vi "Get Component by Unique Name.vi"(0 "Build Analyzer in":refnum<class "Build Analyzer.lvclass">, 5 "Component's Unique Name":string, 11 "error in (no error)":errorcluster) -> (4 "Build Analyzer out":refnum<class "Build Analyzer.lvclass">, 6 "Component":refnum<class "Component.lvclass">, 8 "Found":bool, 15 "error out":errorcluster)   [LabVIEW 2017, in "CL_G3_VIComponentBuilder.lvlib" / "Build Analyzer.lvclass"]
doc: "Returns a component by its unique name."
uses:
  Build Analyzer.lvclass
  Components/Component.lvclass
  Build Analyzer.lvclass/Build Analyzer.ctl
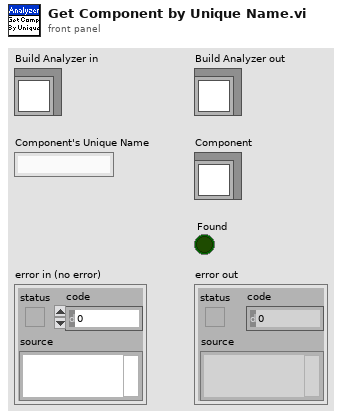
[diagram p1: front panel]
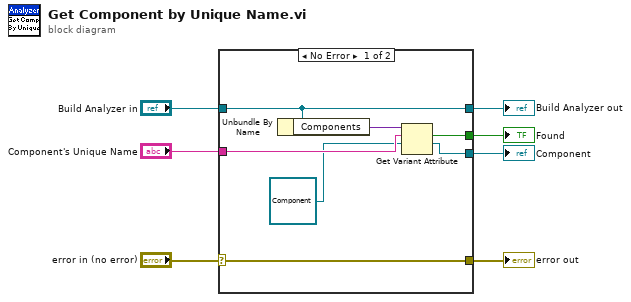
[diagram p0: block diagram]
diagram:
  n1 = case shown="No Error" "error in (no error)" {
    selector: "error in (no error)" -> [w14 w16]
    tunnel: [w14 w16] -> w6
    tunnel: [w13 w15] -> w4
    tunnel: "Build Analyzer in" -> [w13 w15]
    tunnel: "Component's Unique Name" -> [w11 _]
    tunnel: [w9 _] -> w2
    tunnel: [w8 _] -> w1
    frame No Error {
      n2 = Unbundle By Name(w13) -> ("Components"=w12:variant)
      n3 = Get Variant Attribute(Variant=w12, name=w11, default value (empty Variant)=refnum<class "Component.lvclass"> refnum ("Component")) -> (found=w8:bool, value=w9:refnum<class "Component.lvclass">)  [unwired: 1 in, 2 out]
    }
    frame Error {
    }
  }
  "error out" <- w6
  "Build Analyzer out" <- w4
  "Component" <- w2
  "Found" <- w1
